vi "A33ConfigureARB.vi"(0 "VISA resource name":refnum<visa-resource-name>, 1 "ARB Number":i16=1, 2 "Filter (0: OFF)":u16(ring) items=["OFF", "STEP", "NORM"], 3 "Advance mode (0: norm; 1:trig)":u16(ring) items=["Normal", "Triggered"], 5 "Channel (1: Channel1)":u16(ring)=1 items=["Channel1"=1, "Channel2"=2], 7 "Phase (0 deg)":dbl format="%#_12g", 9 "Amplitude (1.0 Vpp)":dbl=1.0 format="%#_12g", 11 "error in (no error)":errorcluster, 12 "DC Offset (0.0 V)":dbl format="%#_12g", 13 "F/SR/P? (0: Frequency)":u16(ring) items=["Frequency", "Sample rate", "Period"], 14 "Freq/SRate/Period (1 Hz)":dbl=1.0 format="%#_12g") -> (4 "VISA resource name out":refnum<visa-resource-name>, 15 "error out":errorcluster)   [LabVIEW 2022 SP3]
doc: "Selects the waveform shape, frequency, amplitude, offset, and phase for a standard waveform."
panel:
  # "Positive # - selects wfm from volatile. Wfm must be loaded first.\nNegative - selects wfm loaded from non-vol memory, wfm must be first loaded into volatile from file!"
  # "Sometimes shows error message - it's ok, it's just\nphase sync command"
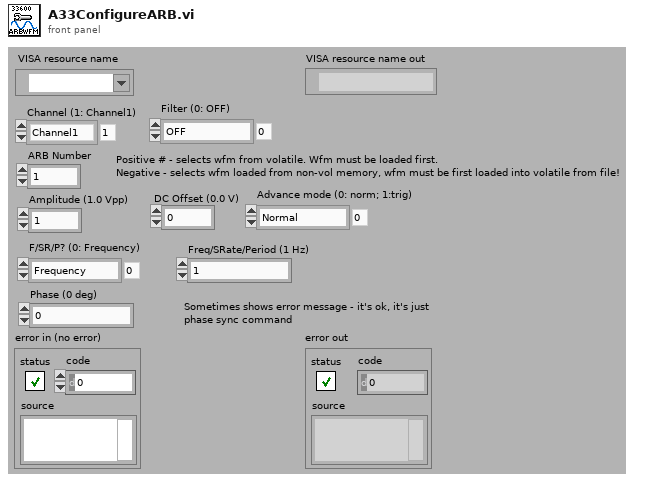
[diagram p1: front panel]
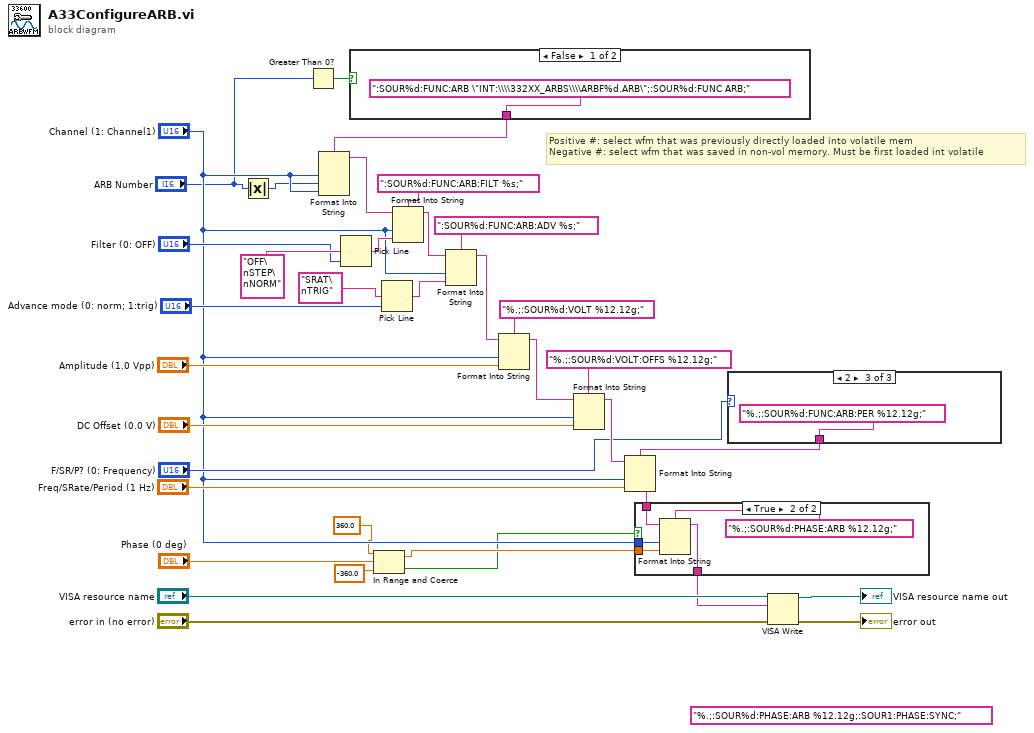
[diagram p0: block diagram]
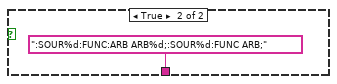
[diagram p3: hidden frame]
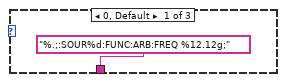
[diagram p4: hidden frame]
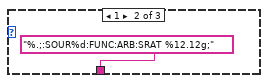
[diagram p5: hidden frame]
diagram:
  (unwired) "%.;:SOUR%d:PHASE:ARB %12.12g;:SOUR1:PHASE:SYNC;"
  # "Positive #: select wfm that was previously directly loaded into volatile mem\nNegative #: select wfm that was saved in non-vol memory. Must be first loaded int volatile"
  n1 = Absolute Value(x="ARB Number") -> (abs(x)=w8:i16)
  n2 = Greater Than 0?(x="ARB Number") -> (x > 0?=w10:bool)
  n3 = Pick Line(multi-line string="OFF\nSTEP\nNORM", line index="Filter (0: OFF)") -> (output string=w22:string)  [unwired: 1 in]
  n4 = case shown="False" w10 {
    tunnel: [":SOUR%d:FUNC:ARB \"INT:\\\\332XX_ARBS\\\\ARBF%d.ARB\";:SOUR%d:FUNC ARB;" ":SOUR%d:FUNC:ARB ARB%d;:SOUR%d:FUNC ARB;"] -> w36
    frame False {
    }
    frame True {
    }
  }
  n5 = Format Into String(format string=w36, "Channel (1: Channel1)", w8, "Channel (1: Channel1)") -> (resulting string=w12:string)  [unwired: 2 in, 1 out]
  n6 = In Range and Coerce(upper limit=360.0, x="Phase (0 deg)", lower limit=-360.0) -> (coerced(x)=w4:dbl, In Range?=w1:bool)
  n7 = Pick Line(multi-line string="SRAT\nTRIG", line index="Advance mode (0: norm; 1:trig)") -> (output string=w18:string)  [unwired: 1 in]
  n8 = Format Into String(format string=":SOUR%d:FUNC:ARB:FILT %s;" ("string"), initial string=w12, "Channel (1: Channel1)", w22) -> (resulting string=w11:string)  [unwired: 1 in, 1 out]
  n9 = Format Into String(format string=":SOUR%d:FUNC:ARB:ADV %s;", initial string=w11, "Channel (1: Channel1)", w18) -> (resulting string=w19:string)  [unwired: 1 in, 1 out]
  n10 = Format Into String(format string="%.;:SOUR%d:VOLT %12.12g;", initial string=w19, "Channel (1: Channel1)", "Amplitude (1.0 Vpp)") -> (resulting string=w14:string)  [unwired: 1 in, 1 out]
  n11 = Format Into String(format string="%.;:SOUR%d:VOLT:OFFS %12.12g;", initial string=w14, "Channel (1: Channel1)", "DC Offset (0.0 V)") -> (resulting string=w31:string)  [unwired: 1 in, 1 out]
  n12 = case shown="2" "F/SR/P? (0: Frequency)" {
    tunnel: ["%.;:SOUR%d:FUNC:ARB:FREQ %12.12g;" "%.;:SOUR%d:FUNC:ARB:SRAT %12.12g;" "%.;:SOUR%d:FUNC:ARB:PER %12.12g;"] -> w25
    frame 0, Default {
    }
    frame 1 {
    }
    frame 2 {
    }
  }
  n13 = Format Into String(format string=w25, initial string=w31, "Channel (1: Channel1)", "Freq/SRate/Period (1 Hz)") -> (resulting string=w7:string)  [unwired: 1 in, 1 out]
  n14 = case shown="True" w1 {
    tunnel: "Channel (1: Channel1)" -> [_ w46]
    tunnel: w7 -> [w42 w45]
    tunnel: [w42 w44] -> w6
    tunnel: w4 -> [_ w43]
    frame False {
    }
    frame True {
      n15 = Format Into String(format string="%.;:SOUR%d:PHASE:ARB %12.12g;", initial string=w45, w46, w43) -> (resulting string=w44:string)  [unwired: 1 in, 1 out]
    }
  }
  n16 = VISA Write(VISA resource name="VISA resource name", write buffer=w6, error in (no error)="error in (no error)") -> (VISA resource name out=→"VISA resource name out":refnum<visa-resource-name>, error out=→"error out":errorcluster)  [unwired: 1 out]
